vi "Sub_Build_MQTT_PubPayload_String.vi"(8 "error in (no error)":errorcluster, 10 "String to be encoded":string="MQIsdp") -> (0 "error out":errorcluster, 2 "UTF8 Byte Array":u8[](array[numeric]) format="%x")   [LabVIEW 2015]
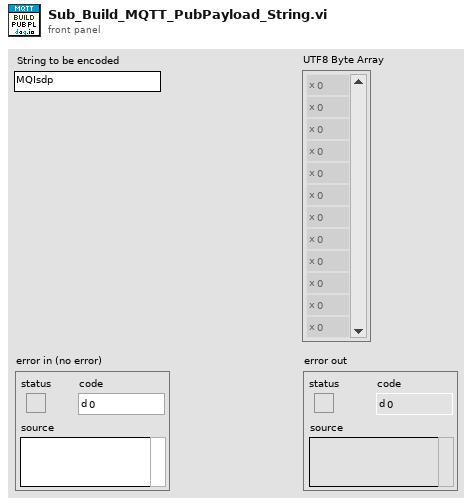
[diagram p1: front panel]
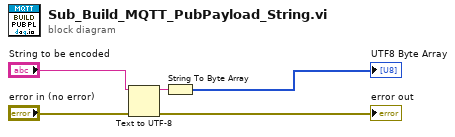
[diagram p0: block diagram]
diagram:
  n1 = Text to UTF-8(8:"error in (no error)", 11:"String to be encoded") -> (0:→"error out":errorcluster, 3:w3:string)  [unwired: 1 in]
  n2 = String To Byte Array(string=w3) -> (unsigned byte array=→"UTF8 Byte Array":u8[])
